vi "4-2 matrice 3xM - matrice max - matrice 100x solfacile.vi"() -> ()   [LabVIEW 2012]
panel:
  out "B(i)":dbl[](array[numeric]) format="%.2f"
  out "A(i)":dbl[](array[numeric]) format="%.2f"
  out "c(i)":dbl[](array[numeric]) format="%.2f"
  out "b(i)":dbl[](array[numeric]) format="%.2f"
  out "a(i)":dbl[](array[numeric]) format="%.2f"
  out "Matrice":dbl[][](array[numeric]) format="%.2f"
  in  "Numero di colonne":i32=4
  # "Realizzare, mediante un generatore di numeri casuali,\n una matrice 3xN [a(i), b(i), c(i) con i che varia  da 0 a N-1] con N impostabile da pannello .\n\n Utilizzando la matrice generata dal SubVi precedente, generare due vettori\n  A(i) e B(i)  [0 <= i <= N-1] con A(i) = Max [a(i),b(i)]  e B(i) = 100*[b(i) + c(N-1-i)]"
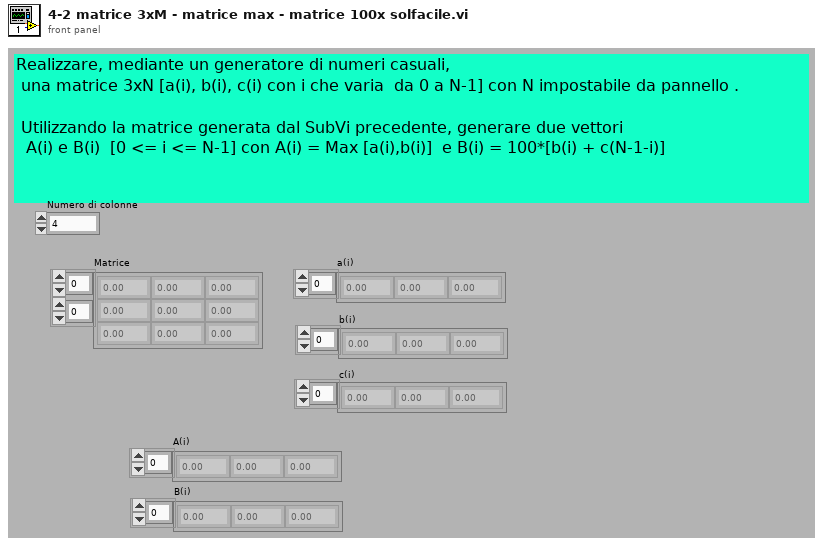
[diagram p1: front panel]
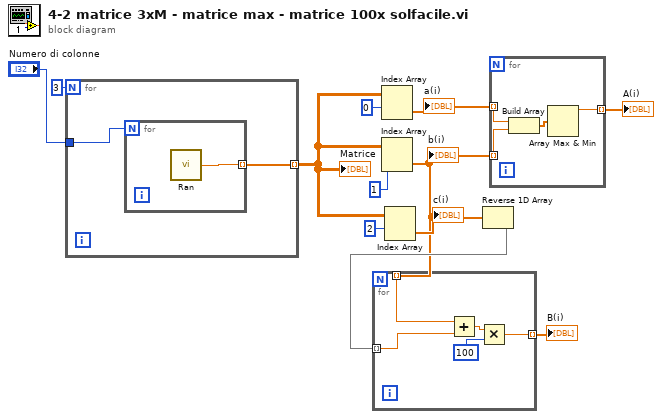
[diagram p0: block diagram]
diagram:
  n1 = for {
    N: 3 -> [_]
    tunnel: "Numero di colonne" -> [w14]
    tunnel: [w13] -> w11 mode=indexing
    n2 = for {
      N: w14 -> [_]
      tunnel: [w15] -> w13 mode=indexing
      n3 = call "Ran.vi"() -> ("out num"=w15:dbl)  [unwired: 5 in]
    }
  }
  "Matrice" <- w11
  n4 = Index Array(array=w11, index (row)=0 ("Array Index")) -> (element=w9:dbl[])  [unwired: 1 in]
  "a(i)" <- w9
  n5 = Index Array(array=w11, index (row)=1 ("Index")) -> (element=w1:dbl[])  [unwired: 1 in]
  "b(i)" <- w1
  n6 = Index Array(array=w11, index (row)=2 ("Index (row)")) -> (element=w8:dbl[])  [unwired: 1 in]
  "c(i)" <- w8
  n7 = Reverse 1D Array(array=w8) -> (reversed array=w4:dbl[])
  n8 = for {
    tunnel: w1 -> [w17] mode=indexing
    tunnel: w4 -> [w16] mode=indexing
    tunnel: [w18] -> w3 mode=indexing
    n9 = Add(x=w17, y=w16) -> (x+y=w20:dbl)
    n10 = Multiply(x=w20, y=100) -> (x*y=w18:dbl)
  }
  "B(i)" <- w3
  n11 = for {
    tunnel: [w24] -> w5 mode=indexing
    tunnel: w9 -> [w21] mode=indexing
    tunnel: w1 -> [w22] mode=indexing
    n12 = Build Array(w21, w22) -> (w23:dbl[])
    n13 = Array Max & Min(array=w23) -> (max value=w24:dbl)  [unwired: 3 out]
  }
  "A(i)" <- w5
